vi "kvCanObjBufSetFlags.vi"(2 "error in (no error)":errorcluster, 3 "Filter Type":bool, 4 "Object Handle":i32, 5 "Channel Handle (input only)":i32) -> (0 "error out":errorcluster, 1 "Channel Handle (output only)":i32)   [LabVIEW 2022 SP3]
doc: "Used to establish whether an Automatic Response object buffer should respond to all message identifiers that match the filter or just RTR message identifiers that match the filter."
uses:
  canlib32.dll
panel:
  # "All Ids"
  # "RTR Ids only"
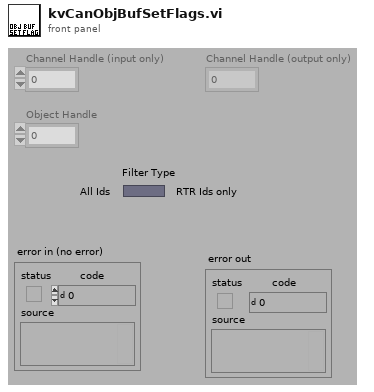
[diagram p1: front panel]
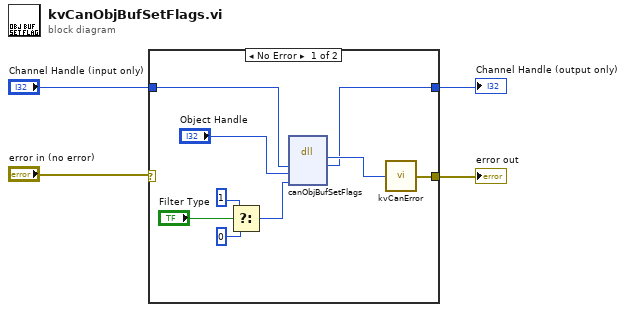
[diagram p0: block diagram]
diagram:
  n1 = case shown="No Error" "error in (no error)" {
    selector: "error in (no error)" -> [_ w14]
    tunnel: "Channel Handle (input only)" -> [w9 w15]
    tunnel: [w5 w15] -> w2
    tunnel: [w13 w14] -> w1
    frame No Error {
      n2 = Select(t=u32 1, s="Filter Type", f=u32 0) -> (s? t:f=w7:u32)
      n3 = dll-call lib="canlib32.dll" fn="canObjBufSetFlags"("channelHandle"=w9, "objectHandle"="Object Handle", "flags"=w7) -> (w6:i32, "channelHandle"=w5:i32)  [unwired: 5 in, 2 out]
      n4 = call "kvCanError.vi"("error code"=w6) -> ("error out"=w13:errorcluster)
    }
    frame Error {
    }
  }
  "Channel Handle (output only)" <- w2
  "error out" <- w1
